vi "PmacProgDownLoadBuffer.vi"(0 "DeviceNumber i32 (0)":i32 min=0, 1 "Program Buffer String":string) -> (2 "Down Load File Path":path, 3 "Down Load Log File Path":path, 4 "Program VI State Cluster":T1={"Program Loaded"=FALSE, "Program Number i32"=1, "Coord Number i32"=1} {"Coord Number i32" min=1 max=8; "Program Number i32" min=1})   [LabVIEW 2020]
doc: "Write Program Buffer to a temporary file then compile and download to PMAC. Down Load File Path and Down Load Log File Path specify the temporary file's name and compile log. If a compile error occurs a modal pop-up panel containing the log is displayed. Program VI State Cluster contains identifies Program Loaded, its Program Number, and Coord Number to run the program in."
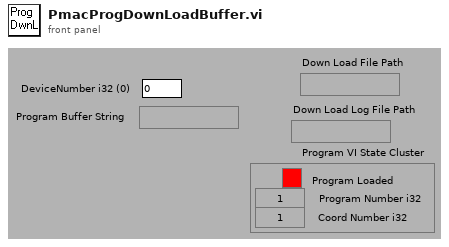
[diagram p1: front panel]
types:
  T1 = cluster{"Program Loaded":bool, "Program Number i32":i32, "Coord Number i32":i32}
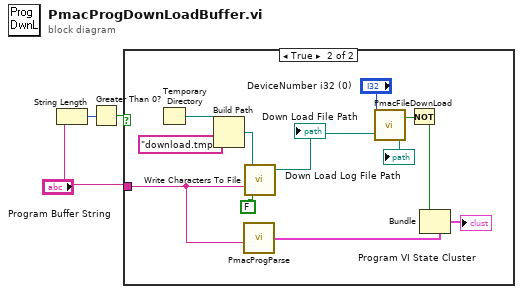
[diagram p0: block diagram]
diagram:
  n1 = String Length(string="Program Buffer String") -> (length=w2:i32)
  n2 = Greater Than 0?(x=w2) -> (x > 0?=w1:bool)
  n3 = case shown="True" w1 {
    tunnel: "Program Buffer String" -> [_ w12]
    frame False {
    }
    frame True {
      n4 = Temporary Directory() -> (w14:path)
      n5 = Build Path(base path=w14, name or relative path="download.tmp") -> (appended path=w5:path)
      n6 = call "PmacProgParse.vi"("Program Buffer String"=w12) -> ("Program VI State Cluster"=w7:T1)
      n7 = call <vilib>:"Write Characters To File.vi"("append to file? (new file:F)"=FALSE, "character string"=w12, "file path (dialog if empty)"=w5) -> ("new file path (Not A Path if cancelled)"=w4:path)  [unwired: 2 out]
      "Down Load File Path" <- w4
      n8 = call "PmacFileDownLoad.vi"("Down Load File Path"=w4, "Device Number i32 (0)"="DeviceNumber i32 (0)") -> ("Down Load Log File Path"=→"Down Load Log File Path":path, "Down Load Error Bool (F)"=w9:bool)
      n9 = Not(x=w9) -> (.not. x?=w8:bool)
      n10 = Bundle(cluster=w7, "Program Loaded"=w8) -> (→"Program VI State Cluster":T1)  [unwired: 2 out]
    }
  }
